vi "Dashboard Main.vi"() -> ()   [LabVIEW 2013]
uses:
  <vilib>/event_ctls.llb/eventvkey.ctl
  <vilib>/Rock Robotics/WPI/Dashboard/WPI_DashboardLogging Global.vi
  <vilib>/Utility/config.llb/Write Key (String).vi
  <vilib>/Utility/config.llb/Write Key (I32).vi
  <vilib>/Utility/config.llb/NI_LVConfig.lvlib
panel:
  in  "Enable Vision":bool
  out "Image Message":string="Timeout in Camera Communications"
  in  "Rec Mode":enum32{"Stop", "Record", "Playback"}(radio)
  in  "Dashboard Tab":T1(tab)
  out "Gear":bool
  in  "AccelRate":dbl=2.5
  out "Distance":dbl
  out "RPM":dbl
  out "Error":bool
  out "Right Motor":dbl(slide) scale=-1.0..1.0 scale format="%#.6g"
  out "StraightDrive":bool
  out "HalfDrive":bool
  out "Left Motor":dbl(slide) scale=-1.0..1.0
  in  "Camera Settings":T2={"Frame Rate"=30, "Compression"=30, "Size"=1} {"Frame Rate" scale=1.0..30.0; "Size" items=["640x480", "320x240", "160x120"]}
  out "MotorSliders R":cluster{"MotorSlide1":dbl, "MotorSlide2":dbl} {"MotorSlide2" scale=-1.0..1.0 scale format="%#_2e"; "MotorSlide1" scale=-1.0..1.0 scale format="%#_2e"}
  out "MotorChart R":cluster{"Numeric":dbl, "Numeric":dbl}(graph)
  out "MotorSliders L":T3 {"MotorSlide4 2" scale=0.0..14.0 scale format="%#_2e"; "MotorSlide2" scale=-1.0..1.0 scale format="%#_2e"; "MotorSlide1" scale=-1.0..1.0 scale format="%#_2e"}
  out "MotorChart L":T4(graph)
  out "Mode":T5(ring)=enum."Auto Disabled"
  out "Camera IP":string
  in  "DB Camera Config":bool
  out "fps":dbl format="%#.1g"
  out "Mbps":dbl format="%#.1g"
  out "Mbps 2":bool
  out "DesiredAngle":dbl
  in  "Test Slider":dbl(slide) scale=0.0..100.0 scale format="%#_3g"
  in  "On/Off":bool caption="Solenoid"
  in  "Test Name":u16(ring) items=["Select the test to run...", "Example Test", "-------------------------------", "List of tests is built in robot code.", "Replace with your own automated tests."]
  in  "Test Tree":string(tree)
  in  "Motor":cluster{"Value":dbl, "Enable":bool} {"Value" scale=-1.0..1.0 scale format="%#_3g"}
  out "Progress":T6 {"Test Progress" scale=0.0..100.0}
  in  "Rev/Fwd":cluster{"Forward":bool, "Reverse":bool}
  in  "Test Ring":u16(ring) items=["Auto", "Fixed indoor", "Fixed outdoor 1", "Fixed outdoor 2", "Fixed fluorescent 1", "Fixed fluorescent 2", "Hold current"]
  in  "Listbox":i32(listbox)
  out "Tree":string(tree)
  out "Errors":T7(array[cluster])
  in  "Reset":bool
  out "Camera Image":T8(plugin-control)
  # "Left"
  # "Front"
  # "Right"
  # "Battery"
  # "Customize by placing controls and indicators here and name to\nmatch Dashboard Variables on robot."
  # "This tab is a great place for autonomous settings and validation.\nCustomize by placing controls and indicators here and name to\nmatch Dashboard Variables on robot."
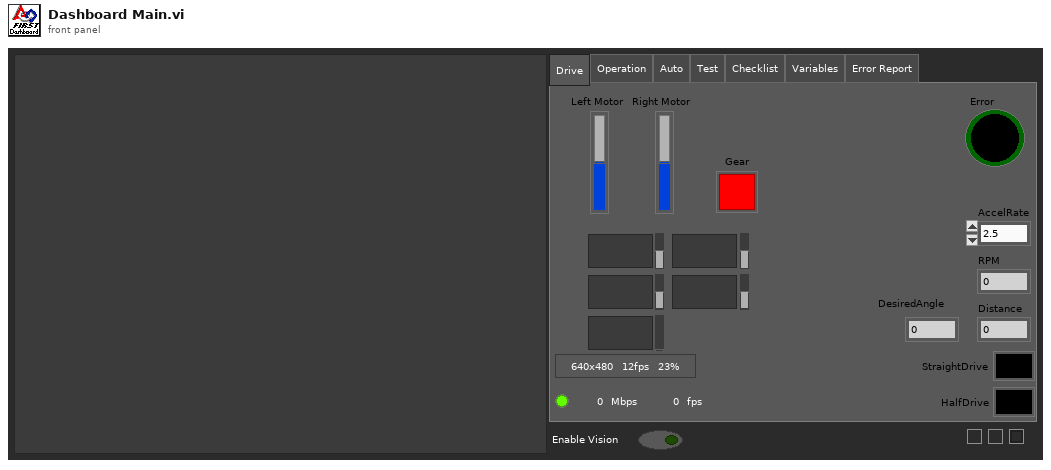
[diagram p1: front panel]
types:
  T1 = enum32{"Drive", "Operation", "Auto", "Test", "Checklist", "Variables", "Error Report"}
  T2 = cluster{"Frame Rate":i32, "Compression":i32, "Size":u16}
  T3 = cluster{"MotorSlide1":dbl, "MotorSlide2":dbl, "MotorSlide4 2":dbl}
  T4 = cluster{"Numeric":dbl, "Numeric":dbl, "Battery":sgl}
  T5 = enum8{"Tele-Op Disabled", "Tele-Op Enabled", "Auto Disabled", "Auto Enabled", "Test Disabled", "Test Enabled", ""}
  T6 = cluster{"Test Progress":u8, "Test Progress Text":string}
  T7 = cluster{"status":bool, "code":i32, "location":string, "source":string}[]
  T8 = typedef "IMAQ Image.ctl" = refnum<image>
  T9 = enum32{"Drive", "Operation", "Auto", "Test", "Checklist", "Variables"}
  T10 = typedef "Image Type" = u32
  T11 = cluster{"Digital Inputs":bool[], "Digital Outputs":bool[]}
  T12 = cluster{"Competition mode":bool, "Robot Link":bool, "Autonomous":bool, "Enabled":bool, "E-Stop":bool, "Simulated":bool, "TestMode":bool, "Docked Window":bool}
  T13 = cluster{"Boolean":bool, "Numeric":i32, "String":string, "String":string}[]
  T14 = typedef "NI_LVConfig.lvlib/Config Data RefNum.ctl" = refnum<k1>
  T15 = typedef "eventvkey.ctl" = enum16{"ASCII", "Enter", "Return", "Shift", "Ctrl", "Alt", "Cmd", "Opt", "Caps", "NumLock", "Clear", "Break", "Up", "Down", "Left", "Right", "Insert", "Delete", "Home", "End", "PageUp", "PageDown", "Escape", "Help", "Pause", "ScrollLock", "F1", "F2", "F3", "F4", "F5", "F6", "F7", "F8", "F9", "F10", "F11", "F12", "F13", "F14", "F15", "F16", "F17", "F18", "F19", "F20", "F21", "F22", "F23", "F24", "Play", "VolumeUp", "VolumeDown", "Mute", "Two Byte Char"}
  T16 = cluster{"Image Size":bool, "Image Type":bool, "Pixel Value":bool, "ROI Information":bool, "Zoom Factor":bool}
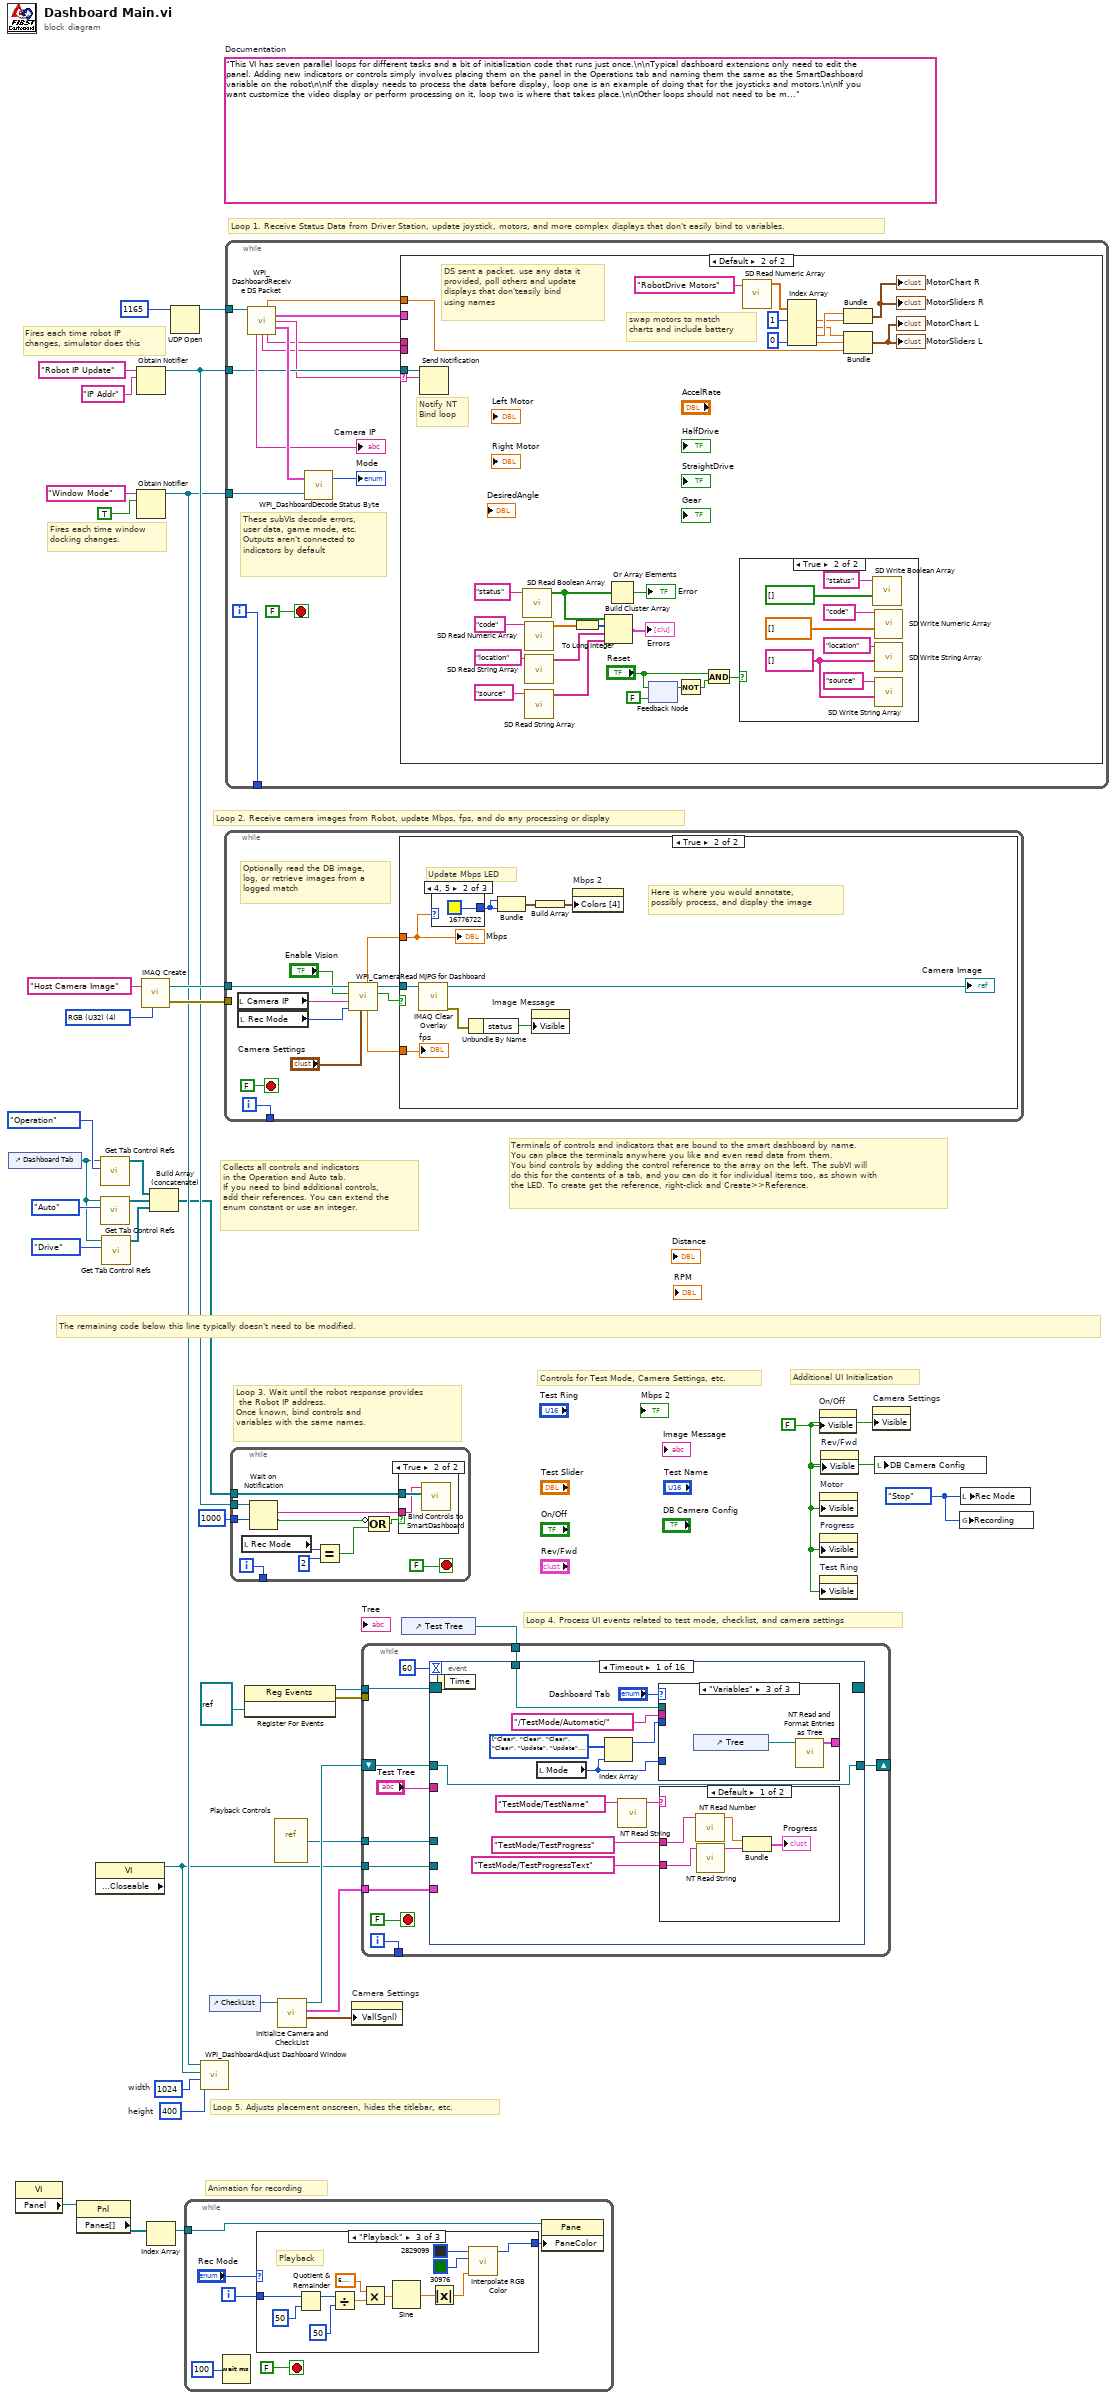
[diagram p0: block diagram]
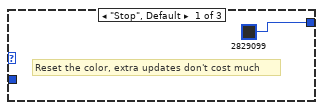
[diagram p2: hidden frame]
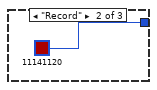
[diagram p3: hidden frame]
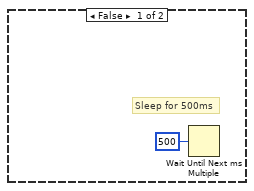
[diagram p5: hidden frame]
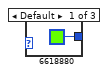
[diagram p6: hidden frame]
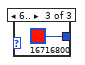
[diagram p7: hidden frame]
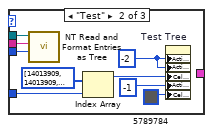
[diagram p9: hidden frame]
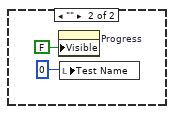
[diagram p10: hidden frame]
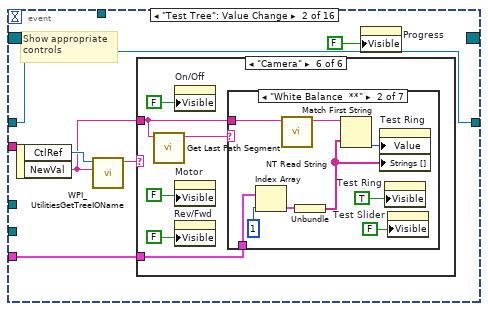
[diagram p11: hidden frame]
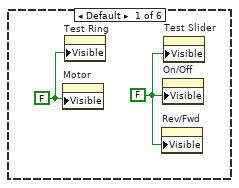
[diagram p12: hidden frame]
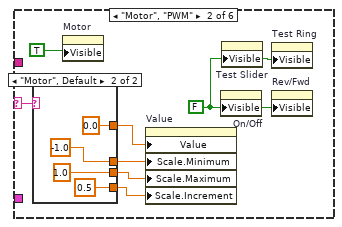
[diagram p13: hidden frame]
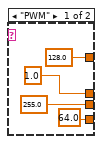
[diagram p14: hidden frame]
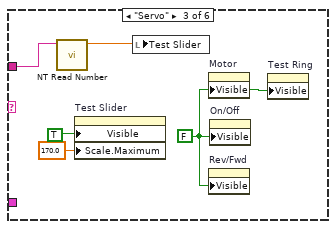
[diagram p15: hidden frame]
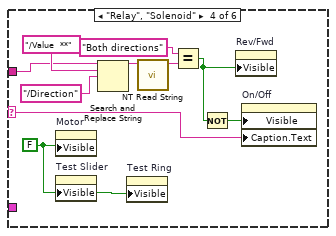
[diagram p16: hidden frame]
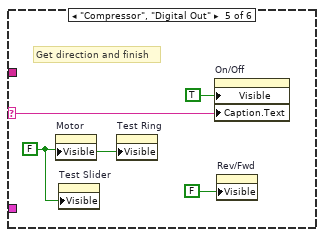
[diagram p17: hidden frame]
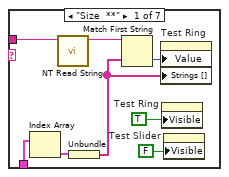
[diagram p18: hidden frame]
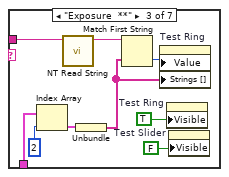
[diagram p19: hidden frame]
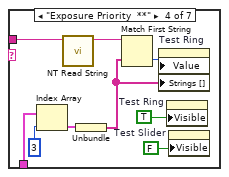
[diagram p20: hidden frame]
diagram:
  w9 = enum32{"Stop", "Record", "Playback"}."Stop" ("Rec Mode")
  w12 = 400  # height
  w13 = 1024  # width
  w26 = FALSE ("Visible")
  (unwired) "This VI has seven parallel loops for different tasks and a bit of initialization code that runs just once.\n\nTypical dashboard extensions only need to edit the panel. Adding new indicators or controls simply involves placing them on the panel in the Operations tab and naming them the same as the SmartDashboard variable on the robot\n\nIf the display needs to process the data before display, loop one is an example of doing that for the joysticks and motors.\n\nIf you want customize the video display or perform processing on it, loop two is where that takes place.\n\nOther loops should not need to be modified. They are pretty standard, and document the task they perform."  # Documentation
  w36 = T10 4 items=["Grayscale (U8)", "Grayscale (I16)", "Grayscale (SGL)", "Complex (CSG)", "RGB (U32)", "HSL (U32)", "RGB (U64)"] ("Image Type")
  # "Controls for Test Mode, Camera Settings, etc."
  # "Additional UI Initialization"
  # "Animation for recording"
  # "Fires each time robot IP\nchanges, simulator does this"
  # "Fires each time window\ndocking changes."
  # "Collects all controls and indicators\nin the Operation and Auto tab.\nIf you need to bind additional controls,\nadd their references. You can extend the\nenum constant or use an integer."
  # "The remaining code below this line typically doesn't need to be modified."
  # "Loop 4. Process UI events related to test mode, checklist, and camera settings"
  # "Terminals of controls and indicators that are bound to the smart dashboard by name.\nYou can place the terminals anywhere you like and even read data from them.\nYou bind controls by adding the control reference to the array on the left. The subVI will\ndo this for the contents of a tab, and you can do it for individual items too, as shown with\nthe LED. To create get the reference, right-click and Create>>Reference."
  # "Loop 3. Wait until the robot response provides\n the Robot IP address.\nOnce known, bind controls and\nvariables with the same names."
  # "Loop 5. Adjusts placement onscreen, hides the titlebar, etc."
  # "Loop 1. Receive Status Data from Driver Station, update joystick, motors, and more complex displays that don't easily bind to variables."
  # "Loop 2. Receive camera images from Robot, update Mbps, fps, and do any processing or display"
  n1 = control-ref of="Dashboard Tab"() -> (w2:refnum<vi>)
  n2 = property class="VI"() -> ("Panel"=w20:refnum<vi>)  [unwired: 2 in, 2 out]
  n3 = property class="Pnl"(reference=w20) -> ("Panes[]"=w21:refnum<vi>[])  [unwired: 1 in, 2 out]
  n4 = property class="VI" props=["Front Panel.Closeable"]() -> (reference out=w8:refnum<vi>)  [unwired: 2 in, 2 out]
  n5 = call <vilib>:"Get Tab Control Refs.vi"("Page Index"=T9."Operation" ("Dashboard Tab"), "TabControl in"=w2) -> ("ControlsOnPage"=w6:refnum<vi>[])  [unwired: 9 in]
  n6 = call <vilib>:"Get Tab Control Refs.vi"("Page Index"=T9."Auto" ("Dashboard Tab"), "TabControl in"=w2) -> ("ControlsOnPage"=w7:refnum<vi>[])  [unwired: 9 in]
  n7 = call <vilib>:"Get Tab Control Refs.vi"("Page Index"=T9."Drive" ("Dashboard Tab"), "TabControl in"=w2) -> ("ControlsOnPage"=w1:refnum<vi>[])  [unwired: 9 in]
  n8 = Obtain Notifier(name (unnamed)="Robot IP Update", notification data type="IP Addr" ("name (unnamed)")) -> (notifier out=w30:refnum<notifier>)  [unwired: 2 in, 2 out]
  n9 = Obtain Notifier(name (unnamed)="Window Mode", notification data type=TRUE) -> (notifier out=w11:refnum<notifier>)  [unwired: 2 in, 2 out]
  n10 = call "IMAQ Create"("Image Name"="Host Camera Image", "Image Type"=w36) -> ("New Image"=w34:T8, "error out"=w33:errorcluster)  [unwired: 2 in, 1 out]
  n11 = Index Array(array=w21) -> (element=w19:refnum<vi>)  [unwired: 1 in]
  n12 = Build Array (concatenate)(w6, w7, w1) -> (w5:refnum<vi>[])
  n13 = UDP Open(11:u16 1165 ("port")) -> (port=w37:refnum<k16>)  [unwired: 2 in, 4 out]
  n14 = while {
    tunnel: w19 -> [w40]
    i -> [w43]
    stop <- FALSE stop-if-true
    n15 = Wait (ms)(milliseconds to wait=u32 100) -> ()  [unwired: 1 out]
    n16 = case shown="\"Playback\"" "Rec Mode" {
      tunnel: w43 -> [_ _ w58]
      tunnel: [u32 2829099 ("Base Color") u32 11141120 ("Target Color") w47] -> w39
      frame "Stop", Default {
        # "Reset the color, extra updates don't cost much"
      }
      frame "Record" {
      }
      frame "Playback" {
        # "Playback"
        n17 = Quotient & Remainder(x=w58, y=u32 50 ("milliseconds to wait")) -> (x-y*floor(x/y)=w54:u32)  [unwired: 1 out]
        n18 = Divide(x=w54, y=u32 50 ("milliseconds to wait")) -> (x/y=w51:dbl)
        n19 = Multiply(x=6.283185307179586, y=w51) -> (x*y=w56:dbl)
        n20 = Sine(x=w56) -> (sin(x)=w55:dbl)
        n21 = Absolute Value(x=w55) -> (abs(x)=w48:dbl)
        n22 = call "Interpolate RGB Color.vi"("Proportion"=w48, "Target Color"=u32 30976, "Base Color"=u32 2829099) -> ("Result Color"=w47:u32)  [unwired: 8 in]
      }
    }
    n23 = property class="Pane"(reference=w40, "PaneColor"=w39) -> ()  [unwired: 1 in, 2 out]
  }
  n24 = call <vilib>:"WPI_DashboardAdjust Dashboard Window.vi"("height"=w12, "width"=w13, "reference in"=w8, "Notifier in"=w11) -> ()  [unwired: 8 in]
  n25 = control-ref of="CheckList"() -> (w10:refnum<vi>)
  n26 = while {
    tunnel: w34 -> [w67]
    tunnel: w33 -> [_]
    tunnel: [w68] -> _
    i -> [w68]
    stop <- FALSE stop-if-true
    # "Optionally read the DB image,\nlog, or retrieve images from a\nlogged match"
    n27 = local read "Camera IP"() -> (w60:string)
    n28 = local read "Rec Mode"() -> (w59:enum32{"Stop", "Record", "Playback"})
    n29 = call <vilib>:"WPI_CameraRead MJPG for Dashboard.vi"("Camera Settings"="Camera Settings", "Rec Mode"=w59, "Camera IP"=w60, "Enable"="Enable Vision", "Refnum in"=w67) -> ("Active"=w64:bool, "Refnum out"=w66:T8, "FPS"=w63:dbl, "Bandwidth (Mbps)"=w62:dbl)  [unwired: 3 in]
    n30 = case shown="True" w64 {
      tunnel: w66 -> [_ w74]
      tunnel: w62 -> [_ w73]
      tunnel: w63 -> [_ w71]
      frame False {
        # "Sleep for 500ms"
        n31 = Wait Until Next ms Multiple(millisecond multiple=u32 500) -> ()  [unwired: 1 out]
      }
      frame True {
        # "Here is where you would annotate,\npossibly process, and display the image"
        # "Update Mbps LED"
        n32 = call "IMAQ Clear Overlay"("Image"=w74) -> ("error out"=w78:errorcluster, "Image Out"=→"Camera Image":T8)  [unwired: 2 in, 7 out]
        n33 = case shown="4, 5" w73 {
          tunnel: [u32 6618880 ("Color Box") u32 16776722 ("Color Box") u32 16716800 ("Color Box")] -> w75
          frame Default {
          }
          frame 4, 5 {
          }
          frame 6.. {
          }
        }
        n34 = Unbundle By Name(w78) -> ("status"=w79:bool)
        n35 = Bundle("Color Box"=w75, "Color Box"=w75) -> (w77:cluster{"Color Box":u32, "Color Box":u32})  [unwired: 1 out]
        n36 = property on="Image Message" class="Str"("Visible"=w79) -> ()  [unwired: 2 in, 2 out]
        n37 = Build Array(w77) -> (w76:cluster{"Color Box":u32, "Color Box":u32}[])
        n38 = property on="Mbps 2" class="Bool (strict)"("Colors [4]"=w76) -> ()  [unwired: 2 in, 2 out]
        "Mbps" <- w73
        "fps" <- w71
      }
    }
  }
  n39 = while {
    tunnel: w37 -> [w93]
    tunnel: w30 -> [w88]
    tunnel: w11 -> [w92]
    tunnel: [w89] -> _
    i -> [w89]
    stop <- FALSE stop-if-true
    # "These subVIs decode errors, user data, game mode, etc.\nOutputs aren't connected to indicators by default"
    n40 = call <vilib>:"WPI_DashboardReceive DS Packet.vi"("Recv Socket"=w93) -> ("Battery"=w83:sgl, "Driver Station"=w84:T11, "Robot IP Address"=w87:string, "Status"=w94:T12, "Camera IP Address"=→"Camera IP":string, "Low Priority User Data"=w86:string, "High Priority User Data"=w85:string)  [unwired: 1 in, 7 out]
    n41 = call <vilib>:"WPI_DashboardDecode Status Byte.vi"("Window Mode Notifier"=w92, "Status"=w94) -> ("Mode"=→"Mode":T5)  [unwired: 1 out]
    n42 = case shown="Default" w87 {
      selector: w87 -> [_ w122]
      tunnel: w88 -> [_ w123]
      tunnel: w86 -> [_ _]
      tunnel: w85 -> [_ _]
      tunnel: w84 -> [_ _]
      tunnel: w83 -> [_ w121]
      frame "0.0.0.0" {
        # "DS not sending packets, or no robot exists yet.\nDon't poll the variables"
      }
      frame Default {
        # "Notify NT\nBind loop"
        # "DS sent a packet. use any data it\nprovided, poll others and update\ndisplays that don'teasily bind\nusing names"
        # "swap motors to match\ncharts and include battery"
        n43 = Send Notification(notification=w122, notifier=w123) -> ()  [unwired: 1 in, 2 out]
        n44 = call <vilib>:"SD Read Boolean Array.vi"("Name"="status") -> ("Boolean Array"=w101:bool[])  [unwired: 8 in, 2 out]
        n45 = call <vilib>:"SD Read Numeric Array.vi"("Name"="code") -> ("Numeric Array"=w100:dbl[])  [unwired: 8 in, 2 out]
        n46 = call <vilib>:"SD Read String Array.vi"("Name"="location") -> ("String Array"=w99:string[])  [unwired: 9 in, 1 out]
        n47 = call <vilib>:"SD Read String Array.vi"("Name"="source") -> ("String Array"=w98:string[])  [unwired: 9 in, 1 out]
        n48 = To Long Integer(number=w100) -> (32bit integer=w106:i32[])
        n49 = Build Cluster Array(w101, w106, w99, w98) -> (→"Errors":T13)
        n50 = Or Array Elements(Boolean array=w101) -> (logical OR=→"Error":bool)
        n51 = feedback #1(FALSE ("Reset")) -> (w109:bool)
        n52 = feedback-in #1("Reset") -> ()
        n53 = Not(x=w109) -> (.not. x?=w108:bool)
        n54 = And(x="Reset", y=w108) -> (x .and. y?=w107:bool)
        n55 = case shown="True" w107 {
          frame False {
          }
          frame True {
            w125 = string[] [] ("String Array")
            n56 = call <vilib>:"SD Write Boolean Array.vi"("Boolean Array"=bool[] [], "Name"="status") -> ()  [unwired: 8 in, 2 out]
            n57 = call <vilib>:"SD Write Numeric Array.vi"("Numeric Array"=dbl[] [], "Name"="code") -> ()  [unwired: 8 in, 2 out]
            n58 = call <vilib>:"SD Write String Array.vi"("String Array"=w125, "Name"="location") -> ()  [unwired: 8 in, 2 out]
            n59 = call <vilib>:"SD Write String Array.vi"("String Array"=w125, "Name"="source") -> ()  [unwired: 8 in, 2 out]
          }
        }
        n60 = call <vilib>:"SD Read Numeric Array.vi"("Name"="RobotDrive Motors") -> ("Numeric Array"=w120:dbl[])  [unwired: 8 in, 2 out]
        n61 = Index Array(array=w120, index #1=1, index #4=0) -> (element #1=w116:dbl, element #2=w115:dbl, element #3=w117:dbl, element #4=w112:dbl)  [unwired: 2 in]
        n62 = Bundle("Numeric"=w117, "Numeric"=w116) -> (→"MotorChart R" →"MotorSliders R":cluster{"Numeric":dbl, "Numeric":dbl})  [unwired: 1 in]
        n63 = Bundle("Numeric"=w115, "Numeric"=w112, "Battery"=w121) -> (→"MotorChart L" →"MotorSliders L":T4)  [unwired: 1 in]
      }
    }
  }
  n64 = while {
    tunnel: w5 -> [w142]
    tunnel: w30 -> [w140]
    tunnel: [w138] -> _
    tunnel: u32 1000 ("milliseconds to wait") -> [w137]
    i -> [w138]
    stop <- FALSE stop-if-true
    n65 = local read "Rec Mode"() -> (w133:enum32{"Stop", "Record", "Playback"})
    n66 = Wait on Notification(notifier=w140, timeout in ms (-1)=w137) -> (notification=w139:string, timed out?=w135:bool)  [unwired: 2 in, 2 out]
    n67 = Equal?(x=w133, y=u16 2 ("Rec Mode")) -> (x = y?=w134:bool)
    n68 = Compound Arithmetic op=OR(invert w135, w134) -> (w136:bool)
    n69 = case shown="True" w136 {
      tunnel: w142 -> [_ w144]
      tunnel: w139 -> [_ w143]
      frame False {
      }
      frame True {
        n70 = call <vilib>:"Bind Controls to SmartDashboard.vi"("Bound Control Refs"=w144, "Server IP Address"=w143) -> ()  [unwired: 10 in]
      }
    }
  }
  n71 = register-events(refnum<vi> refnum) -> (reference out=w17:refnum<event-registration>, error out=w16:errorcluster)  [unwired: 2 in]
  n72 = vi-ref "Playback Controls.vi"() -> (w18:refnum<vi>)
  n73 = call "Initialize Camera and CheckList.vi"("ListBox in"=w10) -> ("Cluster"=w24:cluster{"value":i32, "value":i32, "index":i32}, "Array"=w25:cluster{string[]}[], "File Refnum"=w23:T14)  [unwired: 8 in]
  n74 = property on="Camera Settings" class="Clust (strict)"("Val(Sgnl)"=w24) -> ()  [unwired: 2 in, 2 out]
  n75 = control-ref of="Test Tree"() -> (w22:refnum<vi>)
  n76 = while {
    tunnel: w25 -> [w152]
    shift-right: [w151] -> _
    shift-left: w23 -> [w150]
    tunnel: [w149] -> _
    tunnel: w22 -> [w148]
    tunnel: w18 -> [w147]
    tunnel: w17 -> [w146]
    tunnel: w16 -> [_]
    tunnel: w8 -> [w145]
    i -> [w149]
    stop <- FALSE stop-if-true
    n77 = event shown="[0] Timeout" {
      selector: w146 -> [_ _ _ _ _ _ _ _ _ _ _ _ _ _ _ _]
      dyn-events: [_ _ _ _ _ _ _ _ _ _ _ _ _ w390 _ _] -> _
      timeout: u32 60 ("milliseconds to wait") -> [_ _ _ _ _ _ _ _ _ _ _ _ _ _ _ _]
      tunnel: w148 -> [w162 _ _ _ _ _ _ _ _ _ _ _ _ _ _ _]
      tunnel: "Test Tree" -> [_ _ _ _ _ _ _ _ w359 w367 w369 w373 w381 _ _ _]
      tunnel: w152 -> [_ w186 _ _ _ _ w323 w353 _ _ _ _ _ _ _ _]
      tunnel: [w156 w185 w284 w289 w297 w309 w322 w346 w358 w365 w368 w372 w380 w392 w406 w407] -> w151
      tunnel: w150 -> [w156 w185 w284 w289 w297 w309 w321 w346 w358 w365 w368 w372 w380 w392 w406 w407]
      tunnel: w147 -> [_ _ _ _ _ _ _ _ _ _ _ _ _ w393 _ w410]
      tunnel: w145 -> [_ _ _ _ _ _ _ _ _ _ _ _ _ w388 _ _]
      event Timeout {
        w161 = enum16{"Update", "Clear"}[] [enum."Clear", enum."Clear", enum."Clear", enum."Clear", enum."Update", enum."Update", enum."Clear"] items=["Update", "Clear"]
        n78 = event-data() -> ()  [unwired: 1 in, 1 out]
        n79 = local read "Mode"() -> (w159:T5)
        n80 = Index Array(array=w161, index=w159) -> (element=w160:enum16{"Update", "Clear"})
        n81 = call <vilib>:"NT Read String.vi"("Name"="TestMode/TestName") -> ("String"=w165:string)  [unwired: 9 in, 1 out]
        n82 = case shown="\"Variables\"" "Dashboard Tab" {
          tunnel: w162 -> [_ w175 _]
          tunnel: "/TestMode/Automatic/" ("Name Pattern") -> [_ w174 _]
          tunnel: w160 -> [_ w173 _]
          tunnel: w159 -> [_ w171 _]
          tunnel: [_ _ w177] -> _
          frame "Operation", Default {
          }
          frame "Test" {
            w170 = -2 ("Active Item:Row Number")
            n83 = call <vilib>:"NT Read and Format Entries as Tree.vi"("Operation"=w173, "Name Pattern"=w174, "Tree Refnum"=w175) -> ()  [unwired: 7 in, 2 out]
            n84 = Index Array(array=u32[] [14013909, 14013909, 14013909, 14013909, 14013909, 16777215, 14013909], index=w171) -> (element=w169:u32)
            n85 = property on="Test Tree" class="Tree (strict)"("Active Item Row Number"=w170, "ActiveColNum"=w170, "CellBG"=w169, "Active Item Row Number"=-1 ("Active Item:Row Number"), "CellBG"=u32 5789784 ("Color Box")) -> ()  [unwired: 2 in, 2 out]
          }
          frame "Variables" {
            n86 = control-ref of="Tree"() -> (w176:refnum<vi>)
            n87 = call <vilib>:"NT Read and Format Entries as Tree.vi"("Tree Refnum"=w176) -> ("Formatted Strings"=w177:cluster{"Name":string, "Value":string}[])  [unwired: 9 in, 1 out]
          }
        }
        n88 = case shown="Default" w165 {
          tunnel: "TestMode/TestProgress" ("Name") -> [w179 _]
          tunnel: "TestMode/TestProgressText" ("Name") -> [w178 _]
          frame Default {
            n89 = call <vilib>:"NT Read Number.vi"("Name"=w179) -> ("Numeric"=w180:dbl)  [unwired: 9 in, 1 out]
            n90 = call <vilib>:"NT Read String.vi"("Name"=w178) -> ("String"=w181:string)  [unwired: 9 in, 1 out]
            n91 = Bundle("Numeric"=w180, "String"=w181) -> (→"Progress":cluster{"Numeric":dbl, "String":string})  [unwired: 1 in]
          }
          frame "" {
            n92 = property on="Progress" class="Clust (strict)"("Visible"=FALSE) -> ()  [unwired: 2 in, 2 out]
            n93 = local write "Test Name"(u16 0) -> ()
          }
        }
      }
      event "Test Tree": Value Change {
        # "Show appropriate\ncontrols"
        n94 = event-data() -> ("CtlRef"=w189:refnum<vi>, "NewVal"=w187:string)  [unwired: 1 in]
        n95 = call <vilib>:"WPI_UtilitiesGetTreeIOName.vi"("NewVal"=w187, "TreeControl in"=w189) -> ("I/O Name"=w190:string)  [unwired: 9 in]
        n96 = case shown="\"Camera\"" w190 {
          selector: w190 -> [_ w197 _ w215 w224 _]
          tunnel: w187 -> [_ _ w212 w214 _ w231]
          tunnel: w186 -> [_ _ _ _ _ w230]
          frame Default {
            w192 = FALSE ("Visible")
            w191 = FALSE ("Visible")
            n97 = property on="Motor" class="Clust (strict)"("Visible"=w191) -> ()  [unwired: 2 in, 2 out]
            n98 = property on="Test Ring" class="Ring (strict)"("Visible"=w191) -> ()  [unwired: 2 in, 2 out]
            n99 = property on="Rev/Fwd" class="Clust (strict)"("Visible"=w192) -> ()  [unwired: 2 in, 2 out]
            n100 = property on="On/Off" class="Bool (strict)"("Visible"=w192) -> ()  [unwired: 2 in, 2 out]
            n101 = property on="Test Slider" class="Slide (strict)"("Visible"=w192) -> ()  [unwired: 2 in, 2 out]
          }
          frame "Motor", "PWM" {
            w198 = FALSE ("Visible")
            n102 = case shown="\"Motor\", Default" w197 {
              tunnel: [1.0 ("Value") -1.0 ("Value")] -> w196
              tunnel: [255.0 ("Value") 1.0 ("Value")] -> w195
              tunnel: [128.0 ("Value") 0.0 ("Value")] -> w194
              tunnel: [64.0 ("Value") 0.5 ("Value")] -> w193
              frame "PWM" {
              }
              frame "Motor", Default {
              }
            }
            n103 = property on="Motor" class="Clust (strict)"("Visible"=TRUE) -> ()  [unwired: 2 in, 2 out]
            n104 = property on="Value" class="Slide (strict)"("Value"=w194, "Scale.Minimum"=w196, "Scale.Maximum"=w195, "Scale.Increment"=w193) -> ()  [unwired: 2 in, 2 out]
            n105 = property on="On/Off" class="Bool (strict)"("Visible"=w198) -> ()  [unwired: 2 in, 2 out]
            n106 = property on="Test Slider" class="Slide (strict)"("Visible"=w198) -> ()  [unwired: 2 in, 2 out]
            n107 = property on="Test Ring" class="Ring (strict)"("Visible"=w198) -> ()  [unwired: 2 in, 2 out]
            n108 = property on="Rev/Fwd" class="Clust (strict)"("Visible"=w198) -> ()  [unwired: 2 in, 2 out]
          }
          frame "Servo" {
            w210 = FALSE ("Visible")
            n109 = call <vilib>:"NT Read Number.vi"("Name"=w212) -> ("Numeric"=w211:dbl)  [unwired: 9 in, 1 out]
            n110 = property on="Test Slider" class="Slide (strict)"("Visible"=TRUE, "Scale.Maximum"=170.0 ("Scale.Range:Maximum")) -> ()  [unwired: 2 in, 2 out]
            n111 = local write "Test Slider"(w211) -> ()
            n112 = property on="Motor" class="Clust (strict)"("Visible"=w210) -> ()  [unwired: 2 in, 2 out]
            n113 = property on="Rev/Fwd" class="Clust (strict)"("Visible"=w210) -> ()  [unwired: 2 in, 2 out]
            n114 = property on="On/Off" class="Bool (strict)"("Visible"=w210) -> ()  [unwired: 2 in, 2 out]
            n115 = property on="Test Ring" class="Ring (strict)"("Visible"=w210) -> ()  [unwired: 2 in, 2 out]
          }
          frame "Relay", "Solenoid" {
            w213 = FALSE ("Visible")
            n116 = property on="Motor" class="Clust (strict)"("Visible"=w213) -> ()  [unwired: 2 in, 2 out]
            n117 = property on="Test Slider" class="Slide (strict)"("Visible"=w213) -> ()  [unwired: 2 in, 2 out]
            n118 = Search and Replace String(input string=w214, search string="/Value  **", replace string="/Direction") -> (result string=w220:string)  [unwired: 5 in, 3 out]
            n119 = property on="Test Ring" class="Ring (strict)"("Visible"=w213) -> ()  [unwired: 2 in, 2 out]
            n120 = call <vilib>:"NT Read String.vi"("Name"=w220) -> ("String"=w218:string)  [unwired: 9 in, 1 out]
            n121 = Equal?(x="Both directions", y=w218) -> (x = y?=w216:bool)
            n122 = Not(x=w216) -> (.not. x?=w217:bool)
            n123 = property on="Rev/Fwd" class="Clust (strict)"("Visible"=w216) -> ()  [unwired: 2 in, 2 out]
            n124 = property on="On/Off" class="Bool (strict)"("Visible"=w217, "Caption.Text"=w215) -> ()  [unwired: 2 in, 2 out]
          }
          frame "Compressor", "Digital Out" {
            w223 = FALSE ("Visible")
            # "Get direction and finish"
            n125 = property on="Motor" class="Clust (strict)"("Visible"=w223) -> ()  [unwired: 2 in, 2 out]
            n126 = property on="Test Slider" class="Slide (strict)"("Visible"=w223) -> ()  [unwired: 2 in, 2 out]
            n127 = property on="Test Ring" class="Ring (strict)"("Visible"=w223) -> ()  [unwired: 2 in, 2 out]
            n128 = property on="On/Off" class="Bool (strict)"("Visible"=TRUE, "Caption.Text"=w224) -> ()  [unwired: 2 in, 2 out]
            n129 = property on="Rev/Fwd" class="Clust (strict)"("Visible"=FALSE) -> ()  [unwired: 2 in, 2 out]
          }
          frame "Camera" {
            n130 = call <vilib>:"Get Last Path Segment.vi"("String in"=w231) -> ("String out"=w232:string)  [unwired: 10 in]
            n131 = property on="On/Off" class="Bool (strict)"("Visible"=FALSE) -> ()  [unwired: 2 in, 2 out]
            n132 = property on="Motor" class="Clust (strict)"("Visible"=FALSE) -> ()  [unwired: 2 in, 2 out]
            n133 = property on="Rev/Fwd" class="Clust (strict)"("Visible"=FALSE) -> ()  [unwired: 2 in, 2 out]
            n134 = case shown="\"White Balance  **\"" w232 {
              tunnel: w231 -> [w238 w247 w256 w265 w274 _ w280]
              tunnel: w230 -> [w236 w244 w253 w262 w271 _ _]
              frame "Size  **" {
                n135 = Index Array(array=w236) -> (element=w235:cluster{string[]})  [unwired: 1 in]
                n136 = call <vilib>:"NT Read String.vi"("Name"=w238) -> ("String"=w237:string)  [unwired: 9 in, 1 out]
                n137 = Unbundle(w235) -> (w233:string[])
                n138 = Match First String(2:w233, 3:w237) -> (0:w234:i32)  [unwired: 1 out]
                n139 = property on="Test Ring" class="Ring (strict)"("Value"=w234, "Strings []"=w233) -> ()  [unwired: 2 in, 2 out]
                n140 = property on="Test Ring" class="Ring (strict)"("Visible"=TRUE) -> ()  [unwired: 2 in, 2 out]
                n141 = property on="Test Slider" class="Slide (strict)"("Visible"=FALSE) -> ()  [unwired: 2 in, 2 out]
              }
              frame "White Balance  **" {
                n142 = Index Array(array=w244, index=1) -> (element=w245:cluster{string[]})
                n143 = call <vilib>:"NT Read String.vi"("Name"=w247) -> ("String"=w246:string)  [unwired: 9 in, 1 out]
                n144 = Unbundle(w245) -> (w242:string[])
                n145 = Match First String(2:w242, 3:w246) -> (0:w241:i32)  [unwired: 1 out]
                n146 = property on="Test Ring" class="Ring (strict)"("Value"=w241, "Strings []"=w242) -> ()  [unwired: 2 in, 2 out]
                n147 = property on="Test Ring" class="Ring (strict)"("Visible"=TRUE) -> ()  [unwired: 2 in, 2 out]
                n148 = property on="Test Slider" class="Slide (strict)"("Visible"=FALSE) -> ()  [unwired: 2 in, 2 out]
              }
              frame "Exposure  **" {
                n149 = Index Array(array=w253, index=2) -> (element=w254:cluster{string[]})
                n150 = call <vilib>:"NT Read String.vi"("Name"=w256) -> ("String"=w255:string)  [unwired: 9 in, 1 out]
                n151 = Unbundle(w254) -> (w250:string[])
                n152 = Match First String(2:w250, 3:w255) -> (0:w251:i32)  [unwired: 1 out]
                n153 = property on="Test Ring" class="Ring (strict)"("Value"=w251, "Strings []"=w250) -> ()  [unwired: 2 in, 2 out]
                n154 = property on="Test Ring" class="Ring (strict)"("Visible"=TRUE) -> ()  [unwired: 2 in, 2 out]
                n155 = property on="Test Slider" class="Slide (strict)"("Visible"=FALSE) -> ()  [unwired: 2 in, 2 out]
              }
              frame "Exposure Priority  **" {
                n156 = Index Array(array=w262, index=3) -> (element=w263:cluster{string[]})
                n157 = call <vilib>:"NT Read String.vi"("Name"=w265) -> ("String"=w264:string)  [unwired: 9 in, 1 out]
                n158 = Unbundle(w263) -> (w259:string[])
                n159 = Match First String(2:w259, 3:w264) -> (0:w260:i32)  [unwired: 1 out]
                n160 = property on="Test Ring" class="Ring (strict)"("Value"=w260, "Strings []"=w259) -> ()  [unwired: 2 in, 2 out]
                n161 = property on="Test Ring" class="Ring (strict)"("Visible"=TRUE) -> ()  [unwired: 2 in, 2 out]
                n162 = property on="Test Slider" class="Slide (strict)"("Visible"=FALSE) -> ()  [unwired: 2 in, 2 out]
              }
              frame "Color Enable  **" {
                n163 = Index Array(array=w271, index=4) -> (element=w272:cluster{string[]})
                n164 = call <vilib>:"NT Read String.vi"("Name"=w274) -> ("String"=w273:string)  [unwired: 9 in, 1 out]
                n165 = Unbundle(w272) -> (w268:string[])
                n166 = Match First String(2:w268, 3:w273) -> (0:w269:i32)  [unwired: 1 out]
                n167 = property on="Test Ring" class="Ring (strict)"("Value"=w269, "Strings []"=w268) -> ()  [unwired: 2 in, 2 out]
                n168 = property on="Test Ring" class="Ring (strict)"("Visible"=TRUE) -> ()  [unwired: 2 in, 2 out]
                n169 = property on="Test Slider" class="Slide (strict)"("Visible"=FALSE) -> ()  [unwired: 2 in, 2 out]
              }
              frame Default {
                n170 = property on="Test Ring" class="Ring (strict)"("Visible"=FALSE) -> ()  [unwired: 2 in, 2 out]
                n171 = property on="Test Slider" class="Slide (strict)"("Visible"=FALSE) -> ()  [unwired: 2 in, 2 out]
              }
              frame "Brightness  **", "Color Level  **", "Compression  **", "FPS  **", "Sharpness  **" {
                n172 = call <vilib>:"NT Read Number.vi"("Name"=w280) -> ("Numeric"=w279:dbl)  [unwired: 9 in, 1 out]
                n173 = local write "Test Slider"(w279) -> ()
                n174 = property on="Test Slider" class="Slide (strict)"("Visible"=TRUE, "Scale.Maximum"=100.0 ("Scale.Range:Maximum")) -> ()  [unwired: 2 in, 2 out]
                n175 = property on="Test Ring" class="Ring (strict)"("Visible"=FALSE) -> ()  [unwired: 2 in, 2 out]
              }
            }
          }
        }
        n176 = property on="Progress" class="Clust (strict)"("Visible"=FALSE) -> ()  [unwired: 2 in, 2 out]
      }
      event "Test Name": Mouse Enter {
        # "Populate the ring with the list of tests"
        n177 = event-data() -> ()  [unwired: 1 in, 1 out]
        n178 = call <vilib>:"NT Read String Array.vi"("Name"="TestMode/TestList") -> ("String Array"=w288:string[])  [unwired: 9 in, 1 out]
        n179 = Build Array (concatenate)("Select the test to run...", w288) -> (w287:string[])
        n180 = property on="Test Name" class="Ring (strict)"("Strings []"=w287) -> ()  [unwired: 2 in, 2 out]
      }
      event "Test Name": Value Change {
        w290 = FALSE ("Visible")
        # "Tell the robot the test name to run"
        n181 = event-data() -> ("NewVal"=w294:u16)  [unwired: 1 in]
        n182 = property on="Test Name" class="Ring (strict)"() -> ("Strings []"=w295:string[])  [unwired: 2 in, 2 out]
        n183 = local write "Progress"(T6 {"Test Progress"=0, "Test Progress Text"=""} ("Progress")) -> ()
        n184 = Index Array(array=w295, index=w294) -> (element=w293:string)
        n185 = call <vilib>:"NT Write String.vi"("String"=w293, "Name"="TestMode/TestName") -> ()  [unwired: 9 in, 1 out]
        n186 = property on="Progress" class="Clust (strict)"("Visible"=TRUE) -> ()  [unwired: 2 in, 2 out]
        n187 = property on="Motor" class="Clust (strict)"("Visible"=w290) -> ()  [unwired: 2 in, 2 out]
        n188 = property on="Test Slider" class="Slide (strict)"("Visible"=w290) -> ()  [unwired: 2 in, 2 out]
        n189 = property on="On/Off" class="Bool (strict)"("Visible"=w290) -> ()  [unwired: 2 in, 2 out]
        n190 = property on="Rev/Fwd" class="Clust (strict)"("Visible"=w290) -> ()  [unwired: 2 in, 2 out]
        n191 = property on="Test Ring" class="Ring (strict)"("Visible"=w290) -> ()  [unwired: 2 in, 2 out]
      }
      event "Listbox": Double Click {
        n192 = event-data() -> ("PlatMods.Shift"=w298:bool, "Row"=w300:i32)  [unwired: 1 in]
        n193 = case shown="True" w298 {
          tunnel: w300 -> [w304 _]
          tunnel: 1 -> [w303 _]
          frame False {
            n194 = property on="Listbox" class="LstBox (strict)"() -> ("Item Symbols"=w302:i32[])  [unwired: 2 in, 2 out]
            n195 = Replace Array Subset(array=w302, new element=w303, index=w304) -> (w301:i32[])
            n196 = property on="Listbox" class="LstBox (strict)"("Item Symbols"=w301) -> ()  [unwired: 2 in, 2 out]
          }
          frame True {
            w305 = 0 ("Top Row")
            n197 = property on="Listbox" class="LstBox (strict)"() -> ("Number of Rows"=w307:u32)  [unwired: 2 in, 2 out]
            n198 = Initialize Array(0, w307) -> (w306:i32[])
            n199 = property on="Listbox" class="LstBox (strict)"("Top Row"=w305, "Value"=w305, "Item Symbols"=w306) -> ()  [unwired: 2 in, 2 out]
          }
        }
      }
      event "Listbox": Key Down {
        n200 = event-data() -> ("VKey"=w311:T15)  [unwired: 1 in]
        n201 = case shown="\"Left\", \"Right\"" w311 {
          selector: w311 -> [w316 _]
          tunnel: eventvkey."Left" ("VKey") -> [w314 _]
          frame "Left", "Right" {
            n202 = Equal?(x=w314, y=w316) -> (x = y?=w315:bool)
            n203 = Select(t=0, s=w315, f=1) -> (s? t:f=w317:i32)
            n204 = property on="Listbox" class="LstBox (strict)"() -> ("Item Symbols"=w320:i32[])  [unwired: 2 in, 2 out]
            n205 = Replace Array Subset(array=w320, new element=w317, index="Listbox") -> (w319:i32[])
            n206 = property on="Listbox" class="LstBox (strict)"("Item Symbols"=w319) -> ()  [unwired: 2 in, 2 out]
          }
          frame Default {
          }
        }
      }
      event "DB Camera Config": Value Change {
        n207 = event-data() -> ("NewVal"=w324:bool)  [unwired: 1 in]
        n208 = case shown="False" w324 {
          tunnel: w323 -> [w333 _]
          tunnel: [w326 w344] -> w322
          tunnel: w321 -> [w325 w344]
          frame False {
            w340 = "Camera"
            w343 = FALSE ("Visible")
            n209 = local read "Camera Settings"() -> (w332:T2)
            n210 = Index Array(array=w333) -> (element=w336:cluster{string[]})  [unwired: 1 in]
            n211 = Unbundle(w332) -> ("Frame Rate"=w331:i32, "Compression"=w330:i32, "Size"=w334:u16)
            n212 = Unbundle(w336) -> (w335:string[])
            n213 = Index Array(array=w335, index=w334) -> (element=w329:string)
            n214 = call-poly <vilib>:"Write Key.vi"("section"=w340, "value"=w329, "key"="Size", "refnum"=w325) -> ("refnum out"=w342:T14)  [unwired: 2 in, 5 out]
            n215 = call-poly <vilib>:"Write Key.vi"("section"=w340, "value"=w331, "key"="FrameRate", "refnum"=w342) -> ("refnum out"=w341:T14)  [unwired: 1 in, 6 out]
            n216 = property on="Camera Settings" class="Clust (strict)"("Visible"=w343) -> ()  [unwired: 2 in, 2 out]
            n217 = local write "DB Camera Config"(w343) -> ()
            n218 = call-poly <vilib>:"Write Key.vi"("section"=w340, "value"=w330, "key"="Compression", "refnum"=w341) -> ("refnum out"=w327:T14)  [unwired: 1 in, 6 out]
            n219 = call <vilib>:"Close Config Data.vi"("refnum"=w327) -> ("file path"=w328:path)  [unwired: 2 in, 8 out]
            n220 = call <vilib>:"Open Config Data.vi"("configuration file path"=w328) -> ("refnum"=w326:T14)  [unwired: 8 in, 2 out]
          }
          frame True {
            n221 = property on="Camera Settings" class="Clust (strict)"("Visible"=TRUE) -> ()  [unwired: 2 in, 2 out]
          }
        }
      }
      event "Camera Settings": Value Change {
        n222 = event-data() -> ("NewVal"=w357:T2)  [unwired: 1 in]
        n223 = Index Array(array=w353) -> (element=w352:cluster{string[]})  [unwired: 1 in]
        n224 = Unbundle(w357) -> ("Frame Rate"=w348:i32, "Compression"=w347:i32, "Size"=w350:u16)
        n225 = Unbundle(w352) -> (w351:string[])
        n226 = Index Array(array=w351, index=w350) -> (element=w349:string)
        n227 = Format Into String(format string="%s   %dfps   %d%%", w349, w348, w347) -> (resulting string=w354:string)  [unwired: 2 in, 1 out]
        n228 = Build Array(w354) -> (w355:string[])
        n229 = property on="DB Camera Config" class="Bool (strict)"("Strings [4]"=w355) -> ()  [unwired: 2 in, 2 out]
      }
      event "Motor.Enable": Value Change {
        n230 = event-data() -> ("NewVal"=w363:bool)  [unwired: 1 in]
        n231 = Unbundle("Motor") -> ("Value"=w362:dbl)  [unwired: 1 out]
        n232 = Select(t=w362, s=w363, f=0.0) -> (s? t:f=w360:dbl)
        n233 = call <vilib>:"NT Write Number.vi"("Numeric"=w360, "Name"=w359) -> ()  [unwired: 9 in, 1 out]
      }
      event "Test Slider": Value Change {
        n234 = event-data() -> ("NewVal"=w366:dbl)  [unwired: 1 in]
        n235 = call <vilib>:"NT Write Number.vi"("Numeric"=w366, "Name"=w367) -> ()  [unwired: 9 in, 1 out]
      }
      event "On/Off": Value Change {
        n236 = event-data() -> ("NewVal"=w371:bool)  [unwired: 1 in]
        n237 = Boolean To (0,1)(Boolean=w371) -> (0, 1=w370:i16)
        n238 = call <vilib>:"NT Write Number.vi"("Numeric"=w370, "Name"=w369) -> ()  [unwired: 9 in, 1 out]
      }
      event "Rev/Fwd": Value Change {
        n239 = event-data() -> ("NewVal.Forward"=w379:bool, "NewVal.Reverse"=w378:bool)  [unwired: 1 in]
        n240 = Boolean To (0,1)(Boolean=w379) -> (0, 1=w375:i16)
        n241 = Boolean To (0,1)(Boolean=w378) -> (0, 1=w377:i16)
        n242 = Negate(x=w377) -> (-x=w376:i16)
        n243 = Add(x=w375, y=w376) -> (x+y=w374:i16)
        n244 = call <vilib>:"NT Write Number.vi"("Numeric"=w374, "Name"=w373) -> ()  [unwired: 9 in, 1 out]
      }
      event "Test Ring": Value Change {
        n245 = event-data() -> ("NewVal"=w383:u16)  [unwired: 1 in]
        n246 = property on="Test Ring" class="Ring (strict)"() -> ("Strings []"=w384:string[])  [unwired: 2 in, 2 out]
        n247 = Index Array(array=w384, index=w383) -> (element=w382:string)
        n248 = call <vilib>:"NT Write String.vi"("String"=w382, "Name"=w381) -> ()  [unwired: 9 in, 1 out]
      }
      event "Rec Mode": Value Change {
        # "Update globals for recording mode and path to read log from.\nClear when logging and let NetworkTables set path for vision to\nuse."
        n249 = event-data() -> ("NewVal"=w394:enum32{"Stop", "Record", "Playback"})  [unwired: 1 in]
        n250 = global write "WPI_DashboardLogging Global.vi" "Logging Filename"(path "") -> ()
        n251 = case shown="\"Stop\", \"Record\"" w394 {
          tunnel: w393 -> [_ w396 w404]
          tunnel: [_ _ w403] -> w390
          tunnel: [_ _ w402] -> _
          tunnel: w388 -> [_ _ w400]
          tunnel: cluster{i32, i32} {-250, 170} -> [_ _ w399]
          tunnel: [_ _ T16 {"Image Size"=TRUE, "Image Type"=TRUE, "Pixel Value"=TRUE, "ROI Information"=TRUE, "Zoom Factor"=FALSE} ("Image Information Shown:All Elements")] -> w386
          tunnel: [_ _ TRUE ("Zoom Factor")] -> w385
          frame Default {
          }
          frame "Stop", "Record" {
            # "Place Window too"
            n252 = invoke class="VI" method="FP.Close"(reference=w396) -> (reference out=w395:refnum<vi>)  [unwired: 2 in, 2 out]
            n253 = invoke class="VI" method="Abort VI"(reference=w395) -> ()  [unwired: 2 in, 3 out]
          }
          frame "Playback" {
            n254 = call "Open Playback Panel.vi"("Offset"=w399, "DB VI Ref"=w400, "Playback in"=w404) -> ("Playback out"=w401:refnum<vi>)  [unwired: 8 in]
            n255 = register-events(w401) -> (reference out=w403:refnum<event-registration>, error out=w402:errorcluster)  [unwired: 2 in]
          }
        }
        n256 = global write "WPI_DashboardLogging Global.vi" "Recording"(w394) -> ()
        n257 = property on="Camera Image" class="ImageControl"("Image Information Shown"=w386, "Image Information Visible"=w385) -> ()  [unwired: 2 in, 2 out]
        n258 = call <vilib>:"WPI_DashboardNT Log FieldName Cache.vi"("Operation"=enum16{"Lookup/Add", "Index", "Clear"}."Clear") -> ()  [unwired: 8 in, 3 out]
      }
      event Panel Close {
        w405 = enum32{"Stop", "Record", "Playback"}."Stop" ("Rec Mode")
        n259 = event-data() -> ()  [unwired: 1 in, 4 out]
        n260 = local write "Rec Mode"(w405) -> ()
        n261 = global write "WPI_DashboardLogging Global.vi" "Recording"(w405) -> ()
      }
      event Panel Close {
        # "Abort playback window and ourself"
        n262 = event-data() -> ()  [unwired: 1 in, 4 out]
        n263 = invoke class="VI" method="FP.Close"(reference=w410) -> (reference out=w409:refnum<vi>)  [unwired: 2 in, 2 out]
        n264 = invoke class="VI" method="Abort VI"(reference=w409) -> (error out=w408:errorcluster)  [unwired: 2 in, 2 out]
        n265 = invoke class="VI" method="Abort VI"(error in=w408) -> ()  [unwired: 2 in, 3 out]
      }
    }
  }
  n266 = property on="On/Off" class="Bool (strict)"("Visible"=w26) -> ()  [unwired: 2 in, 2 out]
  n267 = property on="Motor" class="Clust (strict)"("Visible"=w26) -> ()  [unwired: 2 in, 2 out]
  n268 = property on="Progress" class="Clust (strict)"("Visible"=w26) -> ()  [unwired: 2 in, 2 out]
  n269 = property on="Test Ring" class="Ring (strict)"("Visible"=w26) -> ()  [unwired: 2 in, 2 out]
  n270 = property on="Rev/Fwd" class="Clust (strict)"("Visible"=w26) -> ()  [unwired: 2 in, 2 out]
  n271 = property on="Camera Settings" class="Clust (strict)"("Visible"=w26) -> ()  [unwired: 2 in, 2 out]
  n272 = local write "DB Camera Config"(w26) -> ()
  n273 = global write "WPI_DashboardLogging Global.vi" "Recording"(w9) -> ()
  n274 = local write "Rec Mode"(w9) -> ()
